vi "MovingDateTrans.vi"(2 "INPUT":dbl[](array[numeric])) -> (0 "MOVEING COMMAND":string)   [LabVIEW 2016]
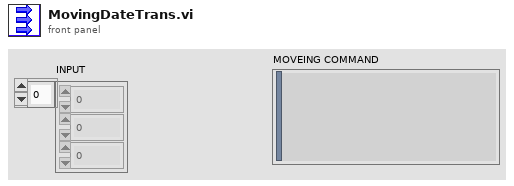
[diagram p1: front panel]
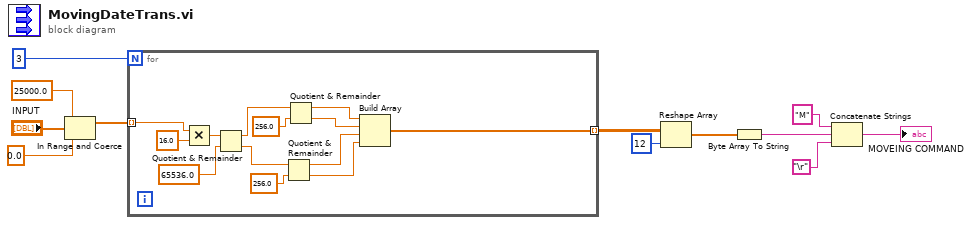
[diagram p0: block diagram]
diagram:
  n1 = In Range and Coerce ("判定范围并强制转换")(upper limit=25000.0 ("上限"), x="INPUT", lower limit=0.0 ("下限")) -> (coerced(x)=w7:dbl[])  [unwired: 1 out]
  n2 = for {
    N: 3 -> [_]
    tunnel: w7 -> [w20] mode=indexing
    tunnel: [w13] -> w4 mode=indexing
    n3 = Multiply(x=w20, y=16.0) -> (x*y=w22:dbl)
    n4 = Quotient & Remainder(x=w22, y=65536.0) -> (x-y*floor(x/y)=w24:dbl, floor(x/y)=w18:dbl)
    n5 = Quotient & Remainder(x=w18, y=256.0) -> (x-y*floor(x/y)=w15:dbl, floor(x/y)=w14:dbl)
    n6 = Quotient & Remainder(x=w24, y=256.0) -> (x-y*floor(x/y)=w17:dbl, floor(x/y)=w16:dbl)
    n7 = Build Array(w17, w16, w15, w14) -> (w13:dbl[])
  }
  n8 = Reshape Array(w4, 12 ("dimension size")) -> (w2:dbl[])
  n9 = Byte Array To String(unsigned byte array=w2) -> (string=w3:string)
  n10 = Concatenate Strings("M" ("string"), w3, "\r") -> (→"MOVEING COMMAND":string)
